vi "Startup Settings.vi"(7 "Name(Global)":string, 8 "error in (no error)":errorcluster, 11 "Tusk in":refnum<class "Tusk.lvclass">) -> (0 "error out":errorcluster, 3 "Tusk out":refnum<class "Tusk.lvclass">)   [LabVIEW 2018, in "Application.lvlib" / "Tusk.lvclass"]
uses:
  Tusk.lvclass
  Tusk.lvclass/Tusk.ctl
  Exceptions Class/VIs/Invalid Name Format.vi
  <vilib>/Utility/error.llb/Trim Whitespace.vi
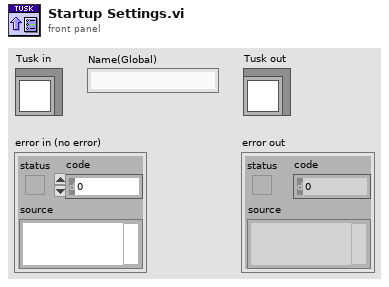
[diagram p1: front panel]
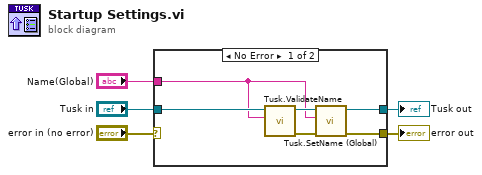
[diagram p0: block diagram]
diagram:
  n1 = case shown="No Error" "error in (no error)" {
    selector: "error in (no error)" -> [_ w13]
    tunnel: [w6 w13] -> w4
    tunnel: [w7 w12] -> w2
    tunnel: "Tusk in" -> [w11 w12]
    tunnel: "Name(Global)" -> [w8 _]
    frame No Error {
      n2 = call "Tusk.ValidateName.vi"("Name"=w8, "Tusk in"=w11) -> ("error out"=w9:errorcluster, "Tusk out"=w10:refnum<class "Tusk.lvclass">)  [unwired: 8 in]
      n3 = call "Tusk.SetName (Global).vi"("error in (no error)"=w9, "Name"=w8, "Tusk in"=w10) -> ("error out"=w6:errorcluster, "Tusk out"=w7:refnum<class "Tusk.lvclass">)  [unwired: 7 in]
    }
    frame Error {
    }
  }
  "error out" <- w4
  "Tusk out" <- w2
